vi "Test Registration API.vi"() -> ()   [LabVIEW 2023]
doc: "Registration API Tester."
uses:
  Data_reg.ctl
  <vilib>/Utility/error.llb/DialogType.ctl
  Registration.lvlib
panel:
  in  "Send Main VI ref":bool
  out "Registration_on":bool
  in  "Data reg 2":T1 {"ЦАП, градС" format="%.3g"; "Тнагр, градС" format="%.3g"; "Q, мл" format="%.3g"; "Рдм, МПа" format="%.3g"; "Тпоп.2, мкс" format="%.3g"; "Тпоп.1, мкс" format="%.3g"; "Тпрод, мкс" format="%.3g"; "Vпл, см3" format="%.1g"; "Рэфф, МПа" format="%.3g"; "dL, мм" format="%.3g"; "R, Ом" format="%.3g"; "Ткд, градС" format="%.3g"; "Ргор, МПа" format="%.2f град.С"; "Рпл2, МПа" format="%.2f град.С"; "Рпл1, МПа" format="%.1g"}
  in  "Show Diagram on Init":bool
  in  "Show Block Diagram":bool
  in  "Stop Module":bool
  in  "Start Module":bool
  in  "Hide Module Panel":bool
  in  "Show Module Panel":bool
  out "Status":string
  out "Module Running?":bool
  # "This VI tests the API for the Module."
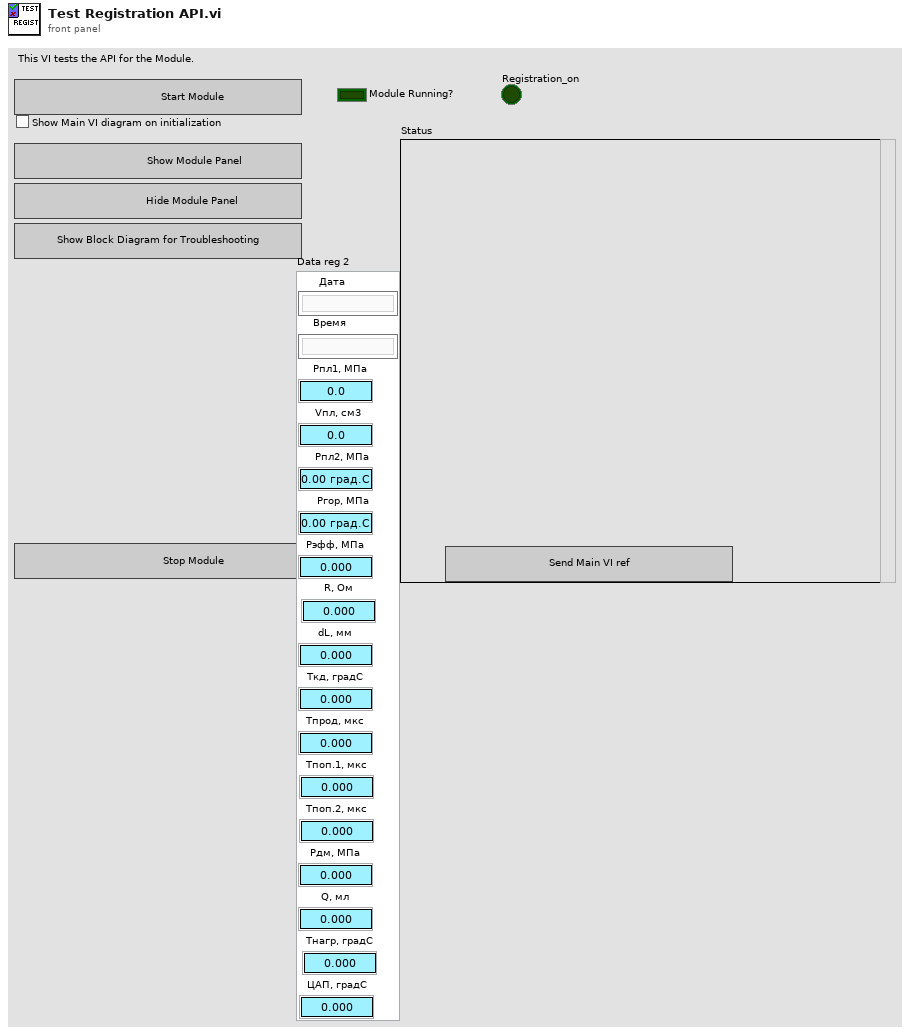
[diagram p1: front panel]
types:
  T1 = typedef "Registration.lvlib/Data_reg.ctl" = cluster{"Дата":string, "Время":string, "Рпл1, МПа":dbl, "Vпл, см3":dbl, "Рпл2, МПа":dbl, "Ргор, МПа":dbl, "Рэфф, МПа":dbl, "R, Ом":dbl, "dL, мм":dbl, "Ткд, градС":dbl, "Тпрод, мкс":dbl, "Тпоп.1, мкс":dbl, "Тпоп.2, мкс":dbl, "Рдм, МПа":dbl, "Q, мл":dbl, "Тнагр, градС":dbl, "ЦАП, градС":dbl}
  T2 = typedef "Registration.lvlib/Broadcast Events--cluster.ctl" = cluster{"Module Did Init":refnum<user-event>, "Status Updated":refnum<user-event>, "Error Reported":refnum<user-event>, "Module Did Stop":refnum<user-event>, "Update Module Execution Status":refnum<user-event>, "Data from Registration":refnum<user-event>, "Get Main VI Reference":refnum<user-event>}
  T3 = typedef "DialogType.ctl" = u16
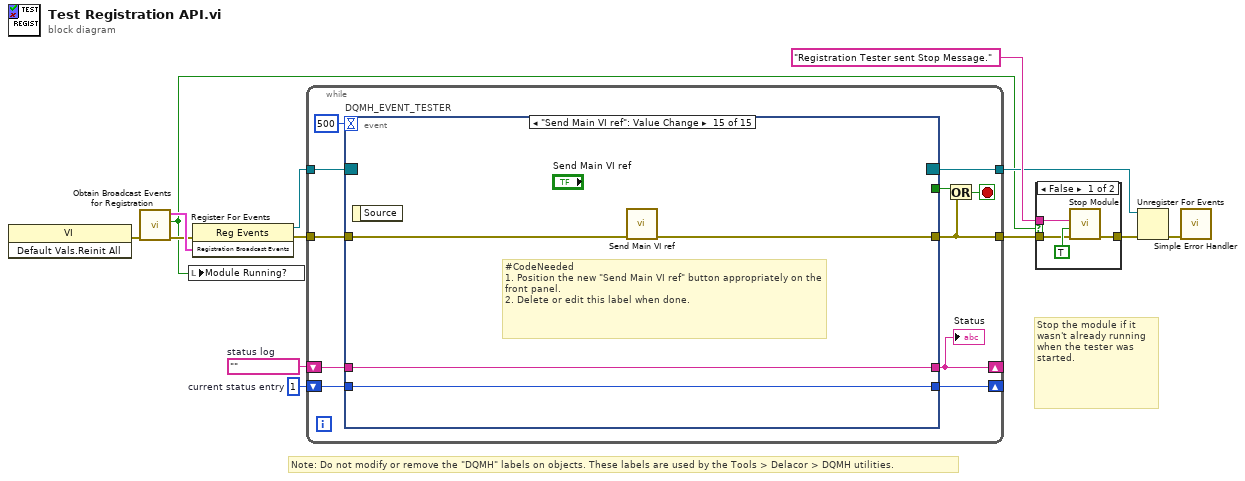
[diagram p0: block diagram]
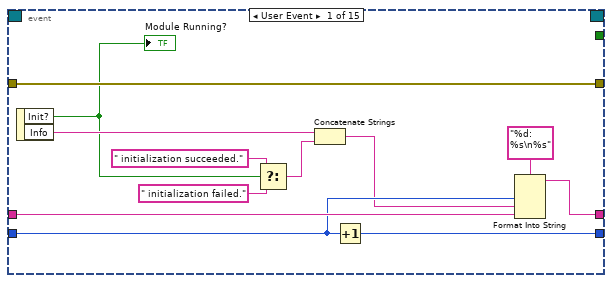
[diagram p3: hidden frame]
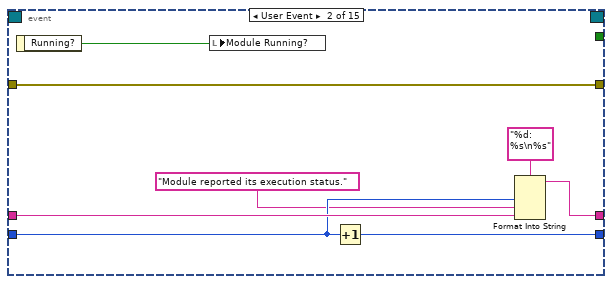
[diagram p4: hidden frame]
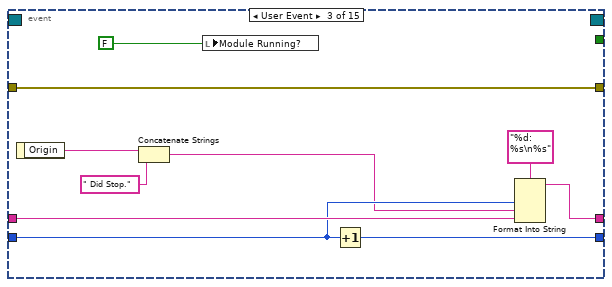
[diagram p5: hidden frame]
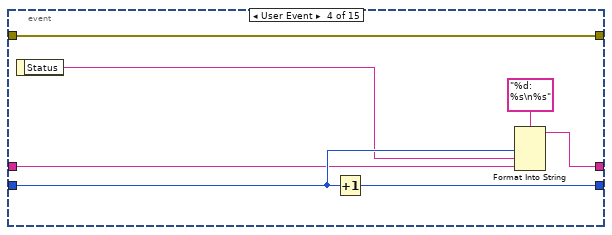
[diagram p6: hidden frame]
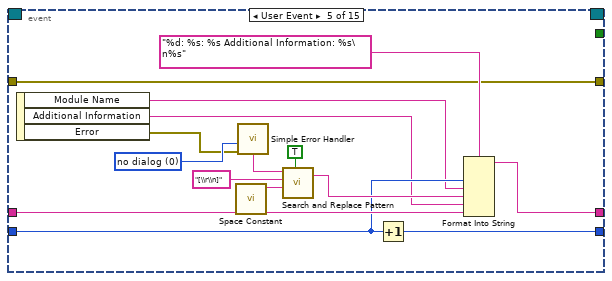
[diagram p7: hidden frame]
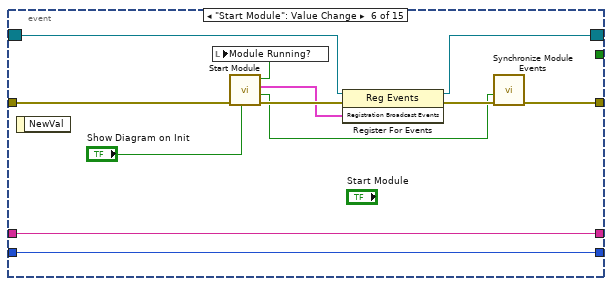
[diagram p8: hidden frame]
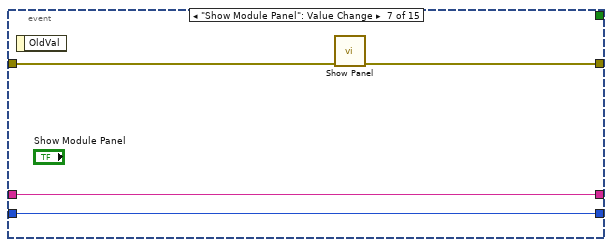
[diagram p9: hidden frame]
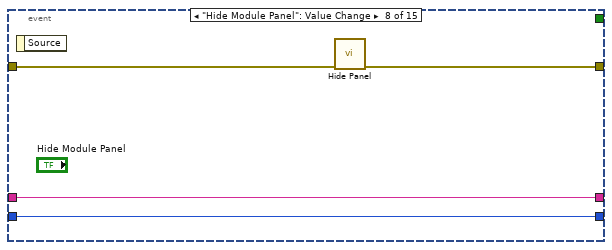
[diagram p10: hidden frame]
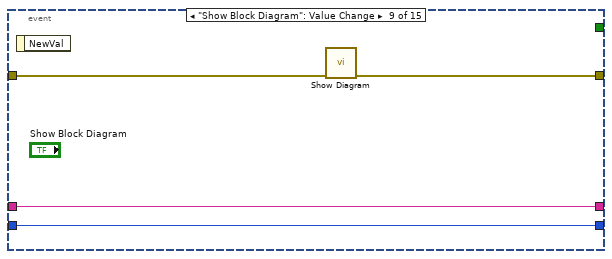
[diagram p11: hidden frame]
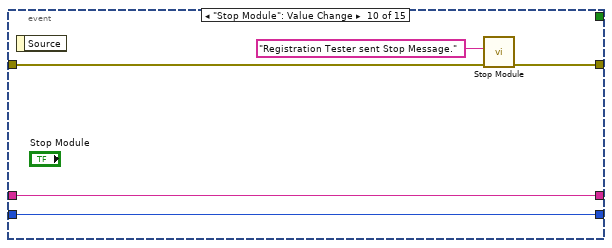
[diagram p12: hidden frame]
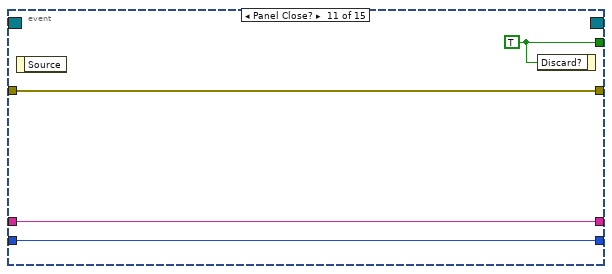
[diagram p13: hidden frame]
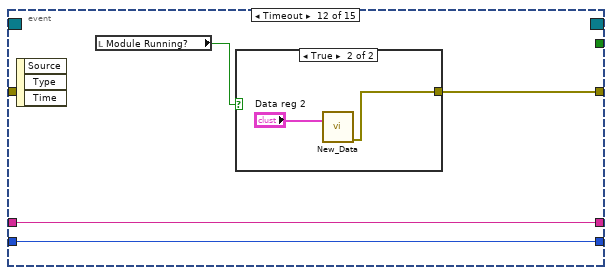
[diagram p14: hidden frame]
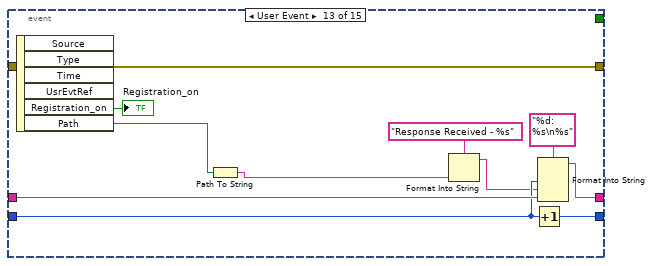
[diagram p16: hidden frame]
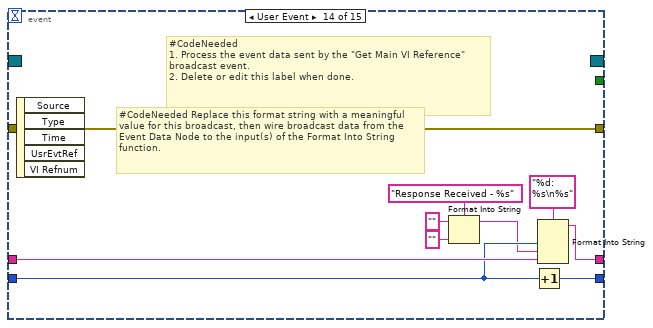
[diagram p17: hidden frame]
diagram:
  w10 = 1  # current status entry
  w11 = ""  # status log
  # "Stop the module if it wasn't already running when the tester was started."
  # "Note: Do not modify or remove the \"DQMH\" labels on objects. These labels are used by the Tools > Delacor > DQMH utilities."
  n1 = invoke class="VI" method="Default Vals.Reinit All"() -> (error out=w5:errorcluster)  [unwired: 3 in, 2 out]
  n2 = call "Obtain Broadcast Events for Registration.vi"("error in"=w5) -> ("error out"=w4:errorcluster, "Already running?"=w3:bool, "Registration Broadcast Events"=w8:T2)  [unwired: 8 in]
  n3 = local write "Module Running?"(w3) -> ()
  n4 = register-events(error in=w4, w8) -> (reference out=w7:refnum<event-registration>, error out=w9:errorcluster)  [unwired: 1 in]
  n5 = while {
    tunnel: w7 -> [w24]
    tunnel: [w15] -> w2
    shift-right: [w19] -> _
    shift-left: w11 -> [w21]
    shift-right: [w20] -> _
    shift-left: w10 -> [w22]
    tunnel: w9 -> [w17]
    tunnel: [w16] -> w6
    stop <- w18 stop-if-true
    n6 = event "DQMH_EVENT_TESTER" shown="[14] \"Send Main VI ref\": Value Change" {
      selector: w24 -> [_ _ _ _ _ w82 _ _ _ _ _ _ _ _ _]
      dyn-events: [_ _ _ _ _ w81 _ _ _ _ _ _ _ _ _] -> w16
      timeout: 500 -> [_ _ _ _ _ _ _ _ _ _ _ _ _ _ _]
      tunnel: [_ _ _ _ _ _ _ _ _ _ w109 _ _ _ _] -> w23
      tunnel: [w36 w38 w45 w55 w65 w80 w92 w96 w97 w103 w106 w111 w126 w136 w137] -> w15
      tunnel: w22 -> [w33 w42 w52 w58 w68 w85 w90 w94 w98 w104 w107 w112 w123 w133 w138]
      tunnel: w21 -> [w34 w43 w53 w57 w69 w86 w91 w95 w99 w105 w108 w113 w125 w135 w139]
      tunnel: [w31 w40 w50 w59 w67 w86 w91 w95 w99 w105 w108 w113 w124 w134 w139] -> w19
      tunnel: [w32 w41 w51 w61 w66 w85 w90 w94 w98 w104 w107 w112 w122 w132 w138] -> w20
      tunnel: w17 -> [w36 w38 w45 w55 w65 w79 w89 w93 w100 w101 w106 _ w126 w136 w140]
      event User Event {
        n7 = event-data() -> ("Init?"=w28:bool, "Info"=w30:string)  [unwired: 1 in]
        "Module Running?" <- w28
        n8 = Select(t=" initialization succeeded.", s=w28, f=" initialization failed.") -> (s? t:f=w25:string)
        n9 = Concatenate Strings(w30, w25) -> (w29:string)
        n10 = Increment(x=w33) -> (x+1=w32:i32)
        n11 = Format Into String(format string="%d: %s\n%s", w33, w29, w34) -> (resulting string=w31:string)  [unwired: 2 in, 1 out]
      }
      event User Event {
        n12 = event-data() -> ("Running?"=w37:bool)  [unwired: 1 in]
        n13 = local write "Module Running?"(w37) -> ()
        n14 = Increment(x=w42) -> (x+1=w41:i32)
        n15 = Format Into String(format string="%d: %s\n%s", w42, "Module reported its execution status.", w43) -> (resulting string=w40:string)  [unwired: 2 in, 1 out]
      }
      event User Event {
        n16 = event-data() -> ("Origin"=w49:string)  [unwired: 1 in]
        n17 = Concatenate Strings(w49, " Did Stop.") -> (w48:string)
        n18 = local write "Module Running?"(FALSE ("Module Did Init?")) -> ()
        n19 = Increment(x=w52) -> (x+1=w51:i32)
        n20 = Format Into String(format string="%d: %s\n%s", w52, w48, w53) -> (resulting string=w50:string)  [unwired: 2 in, 1 out]
      }
      event User Event {
        n21 = event-data() -> ("Status"=w56:string)  [unwired: 1 in]
        n22 = Increment(x=w58) -> (x+1=w61:i32)
        n23 = Format Into String(format string="%d: %s\n%s", w58, w56, w57) -> (resulting string=w59:string)  [unwired: 2 in, 1 out]
      }
      event User Event {
        w70 = T3 0 items=["no dialog", "OK message", "continue or stop message", "OK message + warnings", "continue/stop + warnings"] ("type of dialog (OK msg:1)")
        n24 = event-data() -> ("Module Name"=w64:string, "Additional Information"=w63:string, "Error"=w62:errorcluster)  [unwired: 1 in]
        n25 = call <vilib>:"Space Constant.vi"() -> ("String"=w74:string)
        n26 = call <vilib>:"Simple Error Handler.vi"("type of dialog (OK msg:1)"=w70, "error in (no error)"=w62) -> ("message"=w71:string)  [unwired: 3 in, 4 out]
        n27 = call <vilib>:"Search and Replace Pattern.vi"("string"=w71, "regular expression (\"\")"="[\\r\\n]" ("regular expression (\"\")"), "replace string (\"\")"=w74, "replace all? (F)"=TRUE ("replace all CR/LF with spaces")) -> ("result string"=w72:string)  [unwired: 1 in, 1 out]
        n28 = Increment(x=w68) -> (x+1=w66:i32)
        n29 = Format Into String(format string="%d: %s: %s Additional Information: %s\n%s", w68, w64, w72, w63, w69) -> (resulting string=w67:string)  [unwired: 2 in, 1 out]
      }
      event "Start Module": Value Change {
        n30 = event-data() -> ()  [unwired: 1 in, 1 out]
        n31 = call "Start Module.vi"("Show Main VI Diagram on Init (F)"="Show Diagram on Init", "error in"=w79) -> ("error out"=w87:errorcluster, "Wait for Event Sync?"=w84:bool, "Registration Broadcast Events"=w83:T2, "Module Was Already Running?"=w78:bool)  [unwired: 6 in]
        n32 = local write "Module Running?"(w78) -> ()
        n33 = register-events(reference=w82, error in=w87, w83) -> (reference out=w81:refnum<event-registration>, error out=w88:errorcluster)
        n34 = call "Synchronize Module Events.vi"("error in"=w88, "Wait for Event Sync?"=w84) -> ("error out"=w80:errorcluster)  [unwired: 9 in]
      }
      event "Show Module Panel": Value Change {
        n35 = event-data() -> ()  [unwired: 1 in, 1 out]
        n36 = call "Show Panel.vi"("error in (no error)"=w89) -> ("error out"=w92:errorcluster)  [unwired: 10 in]
      }
      event "Hide Module Panel": Value Change {
        n37 = event-data() -> ()  [unwired: 1 in, 1 out]
        n38 = call "Hide Panel.vi"("error in (no error)"=w93) -> ("error out"=w96:errorcluster)  [unwired: 10 in]
      }
      event "Show Block Diagram": Value Change {
        n39 = event-data() -> ()  [unwired: 1 in, 1 out]
        n40 = call "Show Diagram.vi"("error in (no error)"=w100) -> ("error out"=w97:errorcluster)  [unwired: 10 in]
      }
      event "Stop Module": Value Change {
        n41 = event-data() -> ()  [unwired: 1 in, 1 out]
        n42 = call "Stop Module.vi"("error in"=w101, "Origin"="Registration Tester sent Stop Message.") -> ("error out"=w103:errorcluster)  [unwired: 9 in]
      }
      event Panel Close? {
        w109 = TRUE ("Discard?")
        n43 = event-data() -> ()  [unwired: 1 in, 1 out]
        n44 = event-data("Discard?"=w109) -> ()  [unwired: 1 in, 1 out]
      }
      event Timeout {
        n45 = event-data() -> ()  [unwired: 1 in, 3 out]
        n46 = local read "Module Running?"() -> (w110:bool)
        n47 = case shown="True" w110 {
          tunnel: [_ w114] -> w111
          frame False {
          }
          frame True {
            n48 = call "New_Data.vi"("Data reg"="Data reg 2") -> ("error out"=w114:errorcluster)  [unwired: 10 in]
          }
        }
      }
      event User Event {
        n49 = event-data() -> ("Registration_on"=→"Registration_on":bool, "Path"=w118:path)  [unwired: 1 in, 4 out]
        n50 = Path To String(path=w118) -> (string=w117:string)
        n51 = Format Into String(format string="Response Received - %s", w117) -> (resulting string=w119:string)  [unwired: 2 in, 1 out]
        n52 = Increment(x=w123) -> (x+1=w122:i32)
        n53 = Format Into String(format string="%d: %s\n%s", w123, w119, w125) -> (resulting string=w124:string)  [unwired: 2 in, 1 out]
      }
      event User Event {
        # "#CodeNeeded Replace this format string with a meaningful value for this broadcast, then wire broadcast data from the Event Data Node to the input(s) of the Format Into String function."
        # "#CodeNeeded\n1. Process the event data sent by the \"Get Main VI Reference\" broadcast event.\n2. Delete or edit this label when done."
        n54 = event-data() -> ()  [unwired: 1 in, 5 out]
        n55 = Format Into String(format string="Response Received - %s", initial string="", "" ("input 1")) -> (resulting string=w129:string)  [unwired: 1 in, 1 out]
        n56 = Increment(x=w133) -> (x+1=w132:i32)
        n57 = Format Into String(format string="%d: %s\n%s", w133, w129, w135) -> (resulting string=w134:string)  [unwired: 2 in, 1 out]
      }
      event "Send Main VI ref": Value Change {
        # "#CodeNeeded\n1. Position the new \"Send Main VI ref\" button appropriately on the front panel.\n2. Delete or edit this label when done."
        n58 = event-data() -> ()  [unwired: 1 in, 1 out]
        n59 = call "Send Main VI ref.vi"("error in"=w140) -> ("error out"=w137:errorcluster)  [unwired: 10 in]
      }
    }
    "Status" <- w19
    n60 = Or(x=w23, y=w15) -> (x .or. y?=w18:bool)
  }
  n61 = case shown="False" w3 {
    tunnel: [w144 w145] -> w13
    tunnel: "Registration Tester sent Stop Message." ("Origin") -> [w143 _]
    tunnel: w2 -> [w141 w145]
    frame False {
      n62 = call "Stop Module.vi"("error in"=w141, "Wait for Module to Stop? (F)"=TRUE ("Wait for Module to stop?"), "Origin"=w143) -> ("error out"=w144:errorcluster)  [unwired: 8 in]
    }
    frame True {
    }
  }
  n63 = Unregister For Events(event registration refnum=w6, error in=w13) -> (error out=w1:errorcluster)
  n64 = call <vilib>:"Simple Error Handler.vi"("error in (no error)"=w1) -> ()  [unwired: 4 in, 5 out]
